vi "pack.vi"(8 "error in (no error)":errorcluster, 11 "Dio64FileReader in":refnum<class "Dio64FileReader.lvclass">) -> (0 "error out":errorcluster, 3 "Dio64FileReader out":refnum<class "Dio64FileReader.lvclass">)   [LabVIEW 2011, in "Tools.lvlib" / "Filing.lvlib" / "Dio64FileReader.lvclass"]
uses:
  Dio64FileReader.lvclass
  Dio64FileReader.lvclass/Dio64FileReader.ctl
  FileReader.lvclass
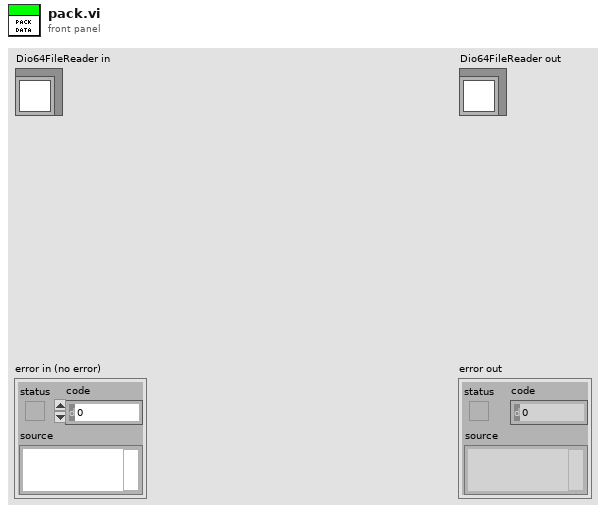
[diagram p1: front panel]
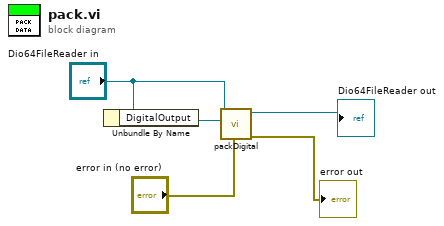
[diagram p0: block diagram]
diagram:
  n1 = Unbundle By Name("Dio64FileReader in") -> ("DigitalOutput"=w1:refnum<class "DigitalOutput.lvclass">)
  n2 = call "packDigital.vi"("error in (no error)"="error in (no error)", "DigitalOutput"=w1, "FileReader in"="Dio64FileReader in") -> ("error out"=→"error out":errorcluster, "FileReader out"=→"Dio64FileReader out":refnum<class "Dio64FileReader.lvclass">)  [unwired: 7 in]
